vi "Read Data From VS Engine.vi"(8 "error in":errorcluster, 9 "Read from VS Engine FIFO":refnum<k33>, 10 "Values Array":dbl[](array[numeric]), 11 "Block Data Ref":T1[](array[typedef]) {"Data Reference" format="%.0x"}) -> (0 "error out":errorcluster, 1 "Read from VS Engine FIFO out":refnum<k33>, 2 "Values Array out":dbl[](array[numeric]), 3 "Block Data Ref out":T1[](array[typedef]) {"Data Reference" format="%.0x"}, 4 "Write Occured":bool)   [LabVIEW 2015, in "Waveform-Processing-Custom-Device Engine.lvlib" / "Inline Async API.lvlib"]
uses:
  Inline Async API.lvlib
  <vilib>/NI Veristand/Custom Device API/Block Data Reference.ctl
  Built/Waveform-Processing-Custom-Device/Waveform-Processing-Custom-Device Engine Windows.llb/Data Reference.ctl
  Built/Waveform-Processing-Custom-Device/c/Waveform-Processing-Custom-Device Engine Pharlap.llb/Global Data Refs.vi
  <vilib>/NI VeriStand/Custom Device API/Custom Device API.lvlib
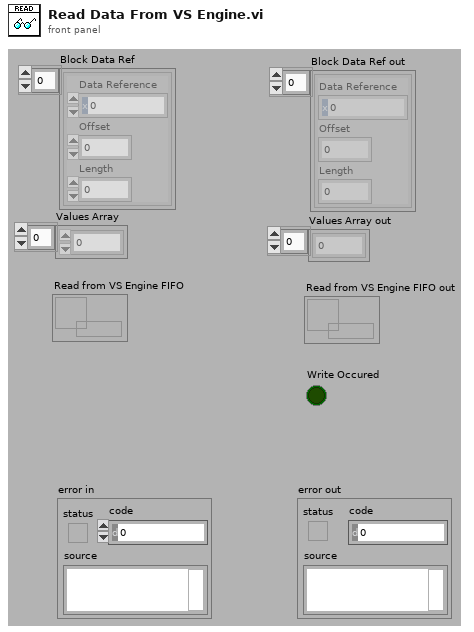
[diagram p1: front panel]
types:
  T1 = typedef "Custom Device API.lvlib/Block Data Reference.ctl" = cluster{"Data Reference":T2, "Offset":u64, "Length":u64}
  T2 = typedef "Custom Device API.lvlib/Data Reference.ctl" = i32
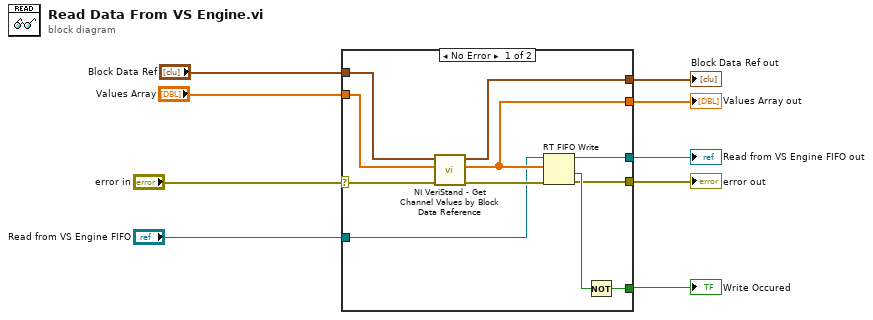
[diagram p0: block diagram]
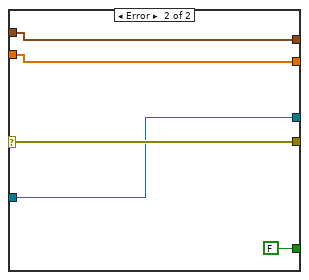
[diagram p2: hidden frame]
diagram:
  n1 = case shown="No Error" "error in" {
    selector: "error in" -> [w17 w25]
    tunnel: [w18 w25] -> w9
    tunnel: [w14 w23] -> w2
    tunnel: [w19 FALSE ("C Read Occured?")] -> w8
    tunnel: [w15 w22] -> w3
    tunnel: "Read from VS Engine FIFO" -> [w13 w21]
    tunnel: "Values Array" -> [w12 w23]
    tunnel: "Block Data Ref" -> [w11 w22]
    tunnel: [w10 w21] -> w1
    frame No Error {
      n2 = call <vilib>:"NI VeriStand - Get Channel Values by Block Data Reference.vi"("error in (no error)"=w17, "Values Array in"=w12, "Block Data Ref"=w11) -> ("error out"=w16:errorcluster, "Values Array out"=w14:dbl[], "Block Data Ref dup"=w15:T1[])  [unwired: 6 in]
      n3 = RT FIFO Write(0:w13, 1:w14, 3:w16) -> (8:w10:refnum<k33>, 10:w20:bool, 11:w18:errorcluster)  [unwired: 2 in, 1 out]
      n4 = Not(x=w20) -> (.not. x?=w19:bool)
    }
    frame Error {
    }
  }
  "error out" <- w9
  "Write Occured" <- w8
  "Block Data Ref out" <- w3
  "Values Array out" <- w2
  "Read from VS Engine FIFO out" <- w1
